vi "Turn.vi"(9 "number of rotations":dbl, 10 "item to rotate":refnum<class>, 11 "Flathead in":refnum<class "Flathead.lvclass">) -> (2 "item rotated":refnum<class>)   [LabVIEW 2023, in "Flathead.lvclass"]
uses:
  Flathead.lvclass
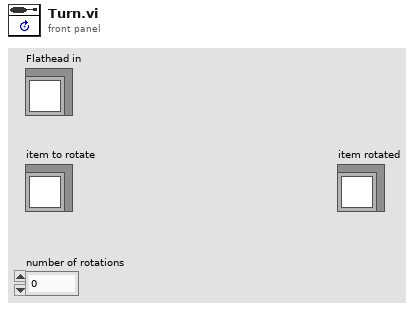
[diagram p1: front panel]
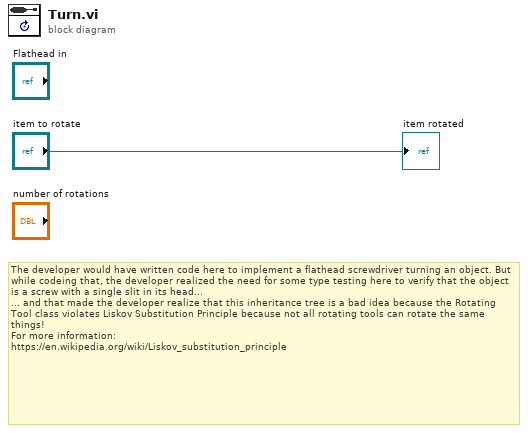
[diagram p0: block diagram]
diagram:
  # "The developer would have written code here to implement a flathead screwdriver turning an object. But while codeing that, the developer realized the need for some type testing here to verify that the object is a screw with a single slit in its head...\n... and that made the developer realize that this inheritance tree is a bad idea because the Rotating Tool class violates Liskov Substitution Principle because not all rotating tools can rotate the same things!\nFor more information:\nhttps://en.wikipedia.org/wiki/Liskov_substitution_principle"
  "item rotated" <- "item to rotate"
